vi "RunningAvg.vi"(10 "Array":dbl[](array[numeric]), 11 "new element":dbl) -> (3 "mean":dbl)   [LabVIEW 2018]
uses:
  <vilib>/Analysis/baseanly.llb/Mean (DBL).vi
  <vilib>/Analysis/NI_AALBase.lvlib
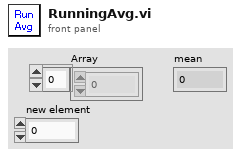
[diagram p1: front panel]
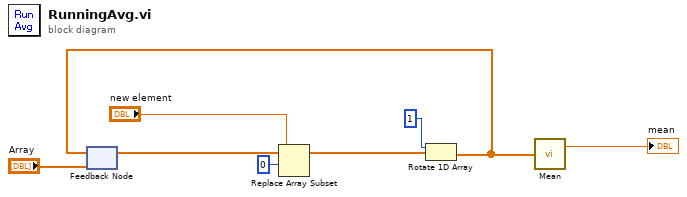
[diagram p0: block diagram]
diagram:
  n1 = feedback #1("Array") -> (w6:dbl[])
  n2 = Replace Array Subset(array=w6, new element="new element", index=0) -> (w5:dbl[])
  n3 = Rotate 1D Array(1:w5, 2:1 ("n")) -> (0:w3:dbl[])
  n4 = feedback-in #1(w3) -> ()
  n5 = call-poly <vilib>:"Mean.vi"("X"=w3) -> ("mean"=→"mean":dbl)  [unwired: 1 out]
